vi "getSlitPosition.vi"(8 "error in (no error)":errorcluster, 10 "SlitType in":T2, 11 "MonoState in":refnum<class "MonoState.lvclass">) -> (0 "error out":errorcluster, 2 "position":T1, 3 "MonoState out":refnum<class "MonoState.lvclass">)   [LabVIEW 2016, in "MonoState.lvclass"]
uses:
  MonoState.lvclass
  Typedefs/SlitType.ctl
  Typedefs/slitPosition.ctl
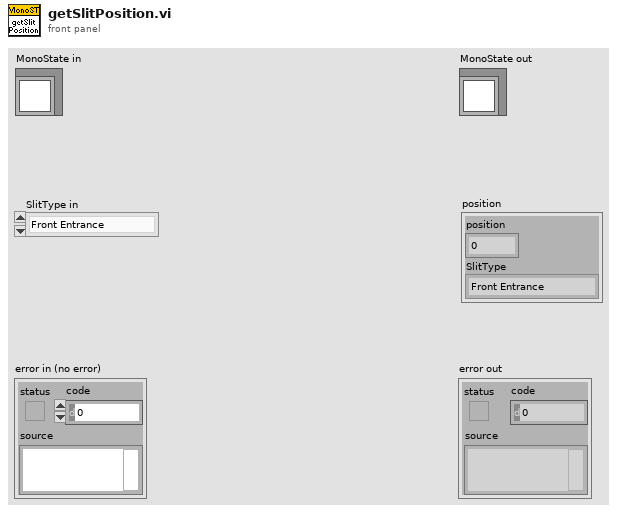
[diagram p1: front panel]
types:
  T1 = typedef "slitPosition.ctl" = cluster{"position":dbl, "SlitType":T2}
  T2 = typedef "SlitType.ctl" = enum16{"Front Entrance", "Side Entrance", "Front Exit", "Side Exit", "First Intermediate", "Second Intermediate"}
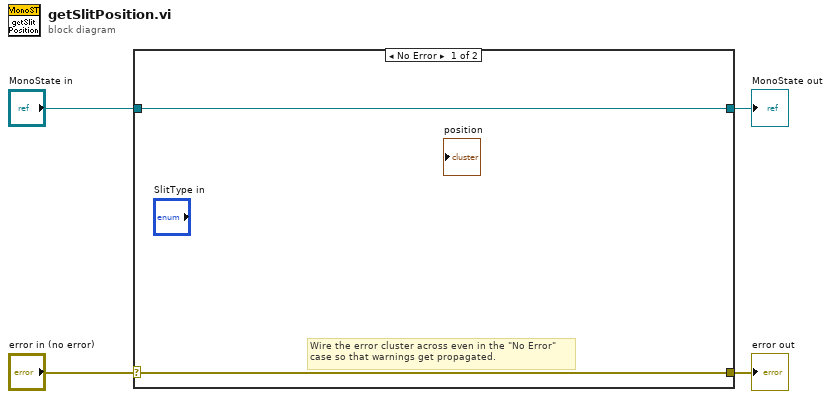
[diagram p0: block diagram]
diagram:
  n1 = case shown="No Error" "error in (no error)" {
    selector: "error in (no error)" -> [w5 w8]
    tunnel: [w5 w8] -> w3
    tunnel: [w6 w7] -> w1
    tunnel: "MonoState in" -> [w6 w7]
    frame No Error {
      # "Wire the error cluster across even in the \"No Error\"\ncase so that warnings get propagated."
    }
    frame Error {
    }
  }
  "error out" <- w3
  "MonoState out" <- w1
